vi "Facade.vi"(0 "Data In":T4=variant(dbl 0.0), 2 "Display State In":T2, 3 "Container State":T3) -> (6 "Data Out":T4=variant(dbl 0.0), 7 "Display State Out":T2, 8 "Action":T1)   [LabVIEW 2021, in "Clock.xctl"]
uses:
  Clock.xctl
  Data.ctl
  <vilib>/_xctls/Container State.ctl
  State.ctl
  <resource>/importtools/Common/Event/NISAST Event.lvclass
  <vilib>/_xctls/Action.ctl
  message.ctl
  <vilib>/_xctls/XControlSupport.lvlib
panel:
  out "hour":dbl(knob) scale=0.0..12.0
  out "minute":dbl(knob) scale=0.0..60.0
  out "second":dbl(knob) scale=0.0..12.0 scale format="%#.0f"
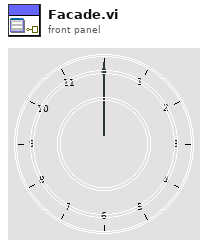
[diagram p1: front panel]
types:
  T1 = typedef "XControlSupport.lvlib/Action.ctl" = cluster{"Data Changed?":bool, "State Changed?":bool, "Action Name":string}
  T2 = typedef "Clock.xctl/State.ctl" = cluster{"Event":refnum<class "NISAST Event.lvclass">, "timer vi":refnum<vi>}
  T3 = typedef "XControlSupport.lvlib/Container State.ctl" = cluster{"Indicator?":bool, "Run Mode?":bool, " Refnum":refnum<vi>}
  T4 = typedef "Clock.xctl/Data.ctl" = variant
  T5 = typedef "Clock.xctl/message.ctl" = cluster{"hour":refnum<vi>, "minute":refnum<vi>, "second":refnum<vi>}
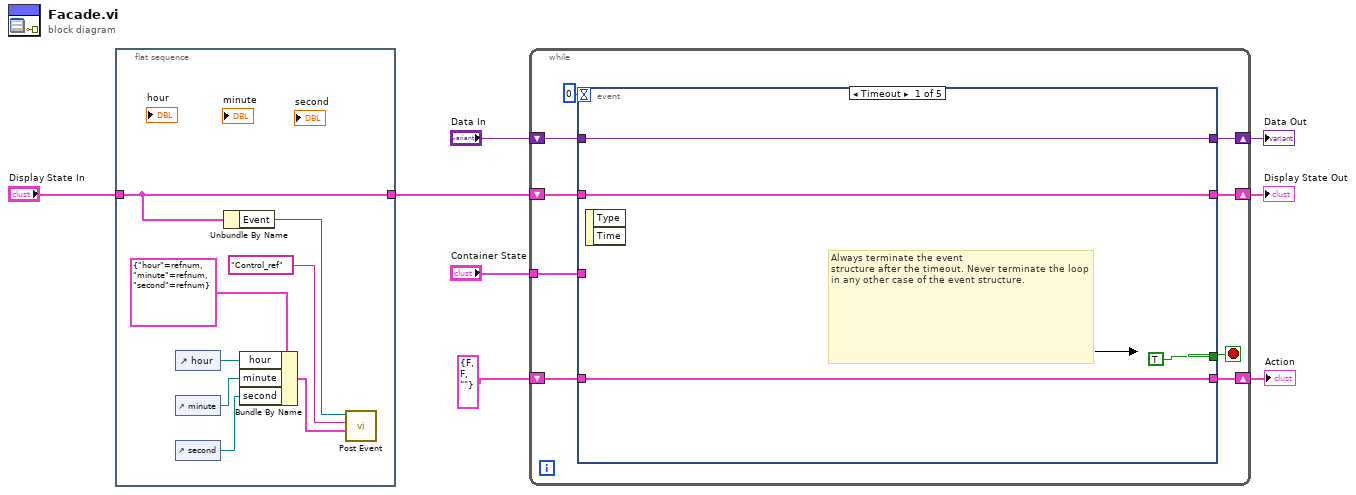
[diagram p0: block diagram]
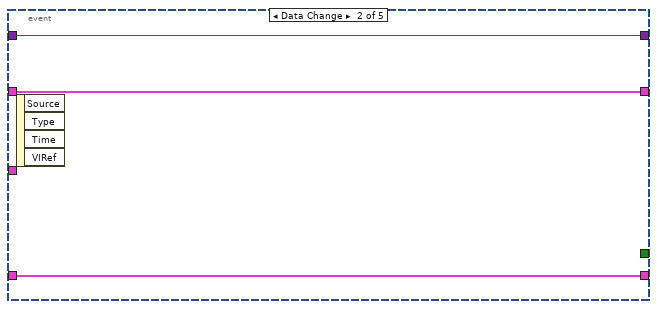
[diagram p2: hidden frame]
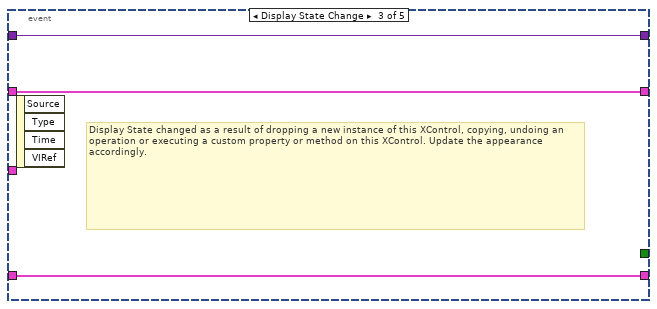
[diagram p3: hidden frame]
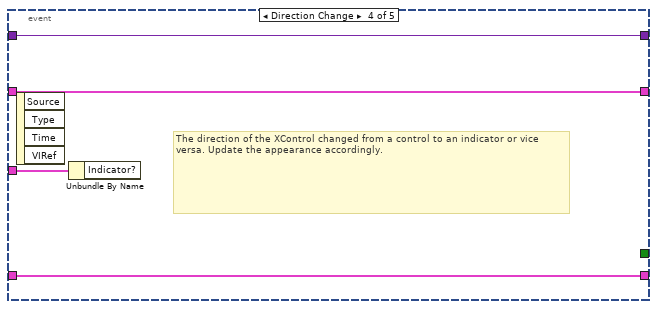
[diagram p4: hidden frame]
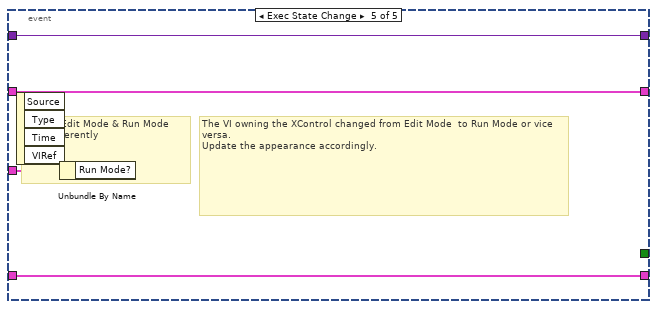
[diagram p5: hidden frame]
diagram:
  n1 = flat-sequence {
    tunnel: "Display State In" -> [w14]
    tunnel: [w14] -> w1
    frame #0 {
      n2 = control-ref of="hour"() -> (w12:refnum<vi>)
      n3 = control-ref of="minute"() -> (w11:refnum<vi>)
      n4 = control-ref of="second"() -> (w10:refnum<vi>)
      n5 = Unbundle By Name(w14) -> ("Event"=w16:refnum<class "NISAST Event.lvclass">)
      n6 = Bundle By Name(cluster=T5 {"hour"=refnum, "minute"=refnum, "second"=refnum} ("message"), "hour"=w12, "minute"=w11, "second"=w10) -> (w9:T5)
      n7 = call-dynamic "Post Event.vi"("Event Data"=w9, "Event Name"="Control_ref", "Event in"=w16) -> ()  [unwired: 7 in, 2 out]
    }
  }
  n8 = while {
    shift-right: [w24] -> w5
    shift-left: w1 -> [w25]
    tunnel: "Container State" -> [w21]
    shift-right: [w19] -> w8
    shift-left: "Data In" -> [w20]
    shift-right: [w17] -> w4
    shift-left: T1 {"Data Changed?"=FALSE, "State Changed?"=FALSE, "Action Name"=""} ("Action") -> [w18]
    stop <- w23 stop-if-true
    n9 = event shown="[0] Timeout" {
      selector: _ -> [_ _ _ _ _]
      dyn-events: _ -> [_ _ _ _ _]
      timeout: 0 -> [_ _ _ _ _]
      tunnel: w25 -> [w27 w31 w35 w38 w42]
      tunnel: [w27 w31 w35 w38 w42] -> w24
      tunnel: [TRUE _ _ _ _] -> w23
      tunnel: w21 -> [_ _ _ w39 w43]
      tunnel: w20 -> [w26 w32 w34 w37 w41]
      tunnel: [w26 w32 w34 w37 w41] -> w19
      tunnel: [w28 w30 w33 w36 w40] -> w17
      tunnel: w18 -> [w28 w30 w33 w36 w40]
      event Timeout {
        # "Always terminate the event\nstructure after the timeout. Never terminate the loop in any other case of the event structure."
        n10 = event-data() -> ()  [unwired: 1 in, 2 out]
      }
      event Data Change {
        n11 = event-data() -> ()  [unwired: 1 in, 4 out]
      }
      event Display State Change {
        # "Display State changed as a result of dropping a new instance of this XControl, copying, undoing an operation or executing a custom property or method on this XControl. Update the appearance accordingly."
        n12 = event-data() -> ()  [unwired: 1 in, 4 out]
      }
      event Direction Change {
        # "The direction of the XControl changed from a control to an indicator or vice versa. Update the appearance accordingly."
        n13 = event-data() -> ()  [unwired: 1 in, 4 out]
        n14 = Unbundle By Name(w39) -> ()  [unwired: 1 out]
      }
      event Exec State Change {
        # "The VI owning the XControl changed from Edit Mode  to Run Mode or vice versa.\nUpdate the appearance accordingly."
        # "Handle Edit Mode & Run Mode\ncase differently"
        n15 = event-data() -> ()  [unwired: 1 in, 4 out]
        n16 = Unbundle By Name(w43) -> ()  [unwired: 1 out]
      }
    }
  }
  "Display State Out" <- w5
  "Data Out" <- w8
  "Action" <- w4
